vi "Get Robot Heading.vi"() -> (0 "Heading":dbl)   [LabVIEW 2011]
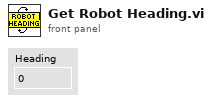
[diagram p1: front panel]
types:
  T1 = typedef "WPI_GyroDevRef.ctl" = cluster{"DevStatus":errorcluster, "Analog Module":T2, "Analog Channel":T3, "Offset":dbl, "Gain (VoltsPerDegree/Second)":dbl}
  T2 = typedef "FPGA_TypedefAnalogModule.ctl" = enum16{"Analog Module 1", "Analog Module 2"}
  T3 = typedef "FPGA_AIChannel.ctl" = enum8{"AI 1", "AI 2", "AI 3", "AI 4", "AI 5", "AI 6", "AI 7", "AI 8", "Invalid"}
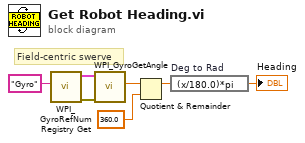
[diagram p0: block diagram]
diagram:
  # "Field-centric swerve"
  n1 = call <vilib>:"WPI_GyroRefNum Registry Get.vi"("refnum name"="Gyro") -> ("error out"=w3:errorcluster, "GyroDevRef"=w1:T1)  [unwired: 9 in]
  n2 = call <vilib>:"WPI_GyroGetAngle.vi"("error in (no error)"=w3, "GyroDevRef"=w1) -> ("Angle"=w5:dbl)  [unwired: 6 in, 3 out]
  n3 = Quotient & Remainder(x=w5, y=360.0) -> (x-y*floor(x/y)=w7:dbl)  [unwired: 1 out]
  n4 = expression code="(x/180.0)*pi" "Deg to Rad"(w7) -> (→"Heading":dbl)
